vi "Globals.vi"() -> ()   [LabVIEW 2021]
panel:
  in  "Send Config over Data port":bool
  in  "Publish Private Config":bool
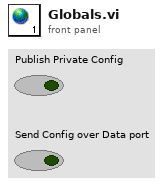
[diagram p1: front panel]
diagram:
